vi "AlliGator Save Phasor Plot Additional Data.vi"(4 "Save only if selected":bool, 5 "Intensity Weighted ? (F)":bool, 6 "Save as...":bool, 7 "Phasor Plot Folder Path (empty)":path, 8 "error in (no error)":errorcluster, 9 "Raw Phasor Plot":T1={"Phasor Plot Name"="", "Raw Phasor Plot"=[], "Phasor Frequency"=160000000.0, "[Decay Metadata]"=[], "Raw Phasor Plot SDV"=[], "Phasor SDV Options"={"Compute Estimated SDV"=FALSE, "# Replicas"=100, "Use Estimated Average Phasor"=FALSE}, "[Calibration Phasor]"=[], "Intensity Array"=[]} {"[Decay Metadata]"."# Folds" min=1; "[Decay Metadata]"."ROI Descriptor"."Contours"."Type" items=["No Selection", "Point", "Line", "Rectangle", "Oval", "Polygon", "Freehand Region", "Annulus", "Unused2", "Unused3", "Broken Line", "Freehand Line", "Rotated Rectangle"]}, 10 "Selected Plot":i32, 11 "Phasor Graph":refnum<vi>) -> (0 "Error Out":errorcluster, 1 "Message":string)   [LabVIEW 2021, in "AlliGator Phasor Graph.lvlib"]
doc: "Save the user-selected Phasor Plot additional data."
uses:
  AlliGator Phasor Graph.lvlib
  AlliGator Raw Phasor Plot Data v5.ctl
  Phasor/Phasor (g, s).ctl
  AlliGator Decay Metadata v3.ctl
  Decay Analysis/Decay Preprocessing/AlliGator Decay Background Subtraction Info.ctl
  Decay Analysis/Decay Preprocessing/AlliGator Baseline Subtraction Method.ctl
  Graphs/XY Graph/XY Graph Plot Shift Parameters.ctl
  Graphs/XY Graph/XY Graph Plot Shift Method.ctl
  Decay Analysis/Decay Preprocessing/AlliGator Decay Extrapolation Parameters.ctl
  Phasor/Phasor Standard Deviation Options.ctl
  Phasor/Calibration Phasor (m, phi).ctl
  Phasor/Phasor.lvlib
  Decay Analysis/Decay Preprocessing/AlliGator Decay Preprocessing.lvlib
  Graphs/XY Graph/XY Graph Add-Ons.lvlib
panel:
  # "see the AlliGator License on the block diagram (Ctrl+E or Window:Show Block Diagram)"
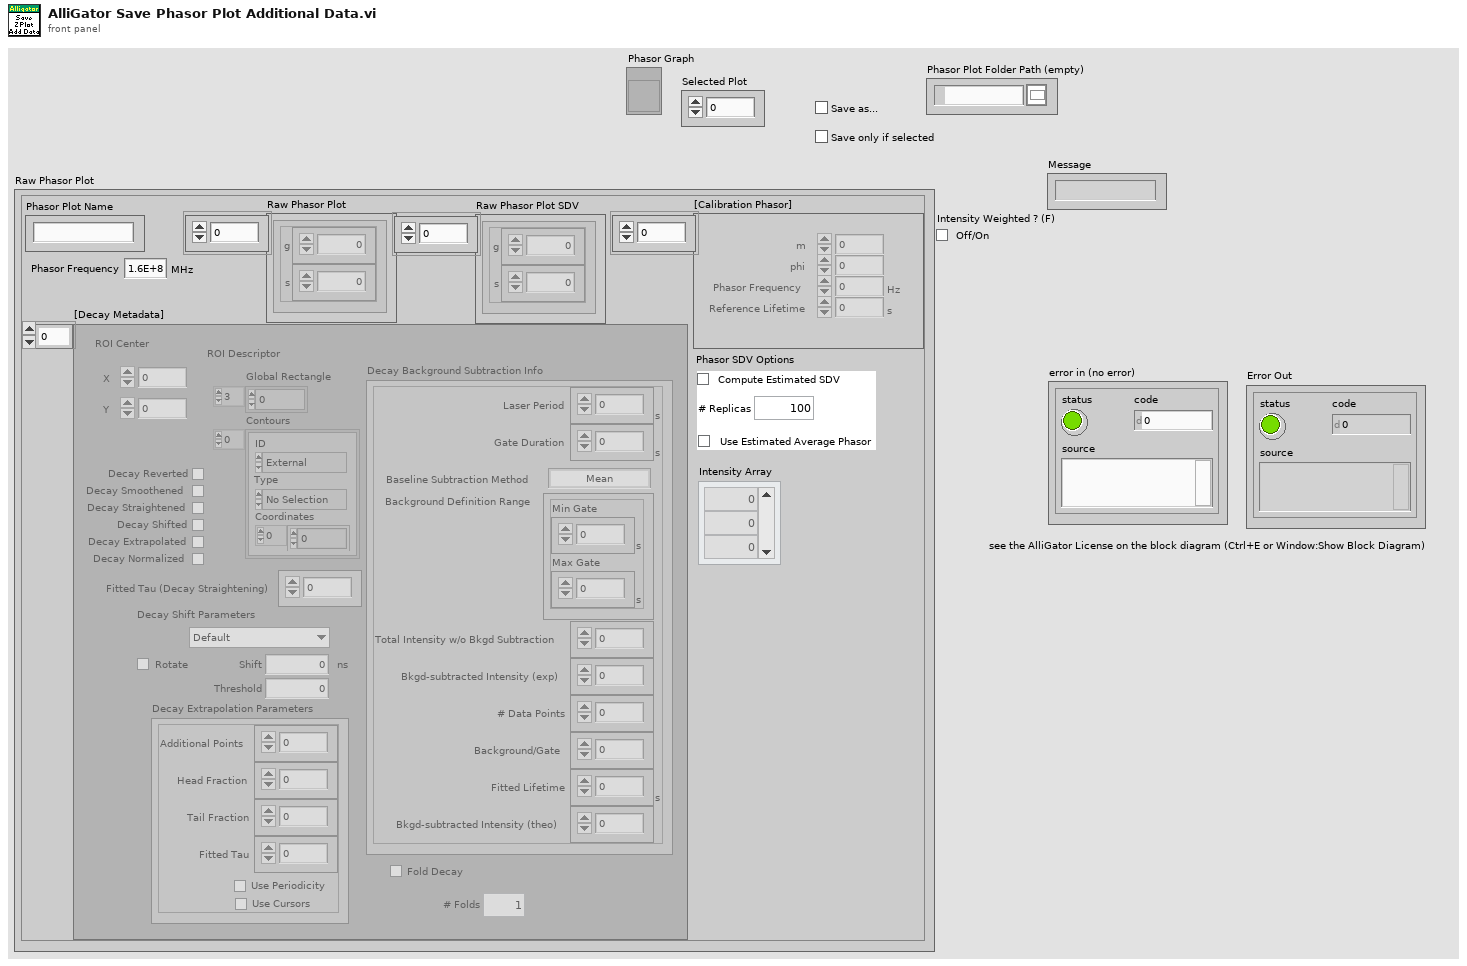
[diagram p1: front panel]
types:
  T1 = typedef "AlliGator Phasor Graph.lvlib/AlliGator Raw Phasor Plot Data v5.ctl" = cluster{"Phasor Plot Name":string, "Raw Phasor Plot":T2[], "Phasor Frequency":dbl[unit], "[Decay Metadata]":T3[], "Raw Phasor Plot SDV":T2[], "Phasor SDV Options":T10, "[Calibration Phasor]":T11[], "Intensity Array":dbl[]}
  T2 = typedef "Phasor.lvlib/Phasor (g, s).ctl" = cluster{"g":dbl, "s":dbl}
  T3 = typedef "AlliGator Phasor Graph.lvlib/AlliGator Decay Metadata v3.ctl" = cluster{"ROI Descriptor":T4, "ROI Center":cluster{"X":i32, "Y":i32}, "Decay Background Subtraction Info":T5, "Decay Reverted":bool, "Decay Smoothened":bool, "Decay Straightened":bool, "Fitted Tau (Decay Straightening)":dbl, "Decay Shift Parameters":T7, "Decay Shifted":bool, "Decay Extrapolated":bool, "Decay Extrapolation Parameters":T9, "Decay Normalized":bool, "Fold Decay":bool, "# Folds":u32}
  T4 = typedef "ROI Descriptor" = cluster{"Global Rectangle":i32[], "Contours":cluster{"ID":enum32{"External", "Internal"}, "Type":u32, "Coordinates":i32[]}[]}
  T5 = typedef "AlliGator Decay Preprocessing.lvlib/AlliGator Decay Background Subtraction Info.ctl" = cluster{"Laser Period":dbl[unit], "Gate Duration":dbl[unit], "Baseline Subtraction Method":T6, "Background Definition Range":cluster{"Min Gate":dbl[unit], "Max Gate":dbl[unit]}, "Total Intensity w/o Bkgd Subtraction":dbl, "Bkgd-subtracted Intensity (exp)":dbl, "# Data Points":i32, "Background/Gate":dbl, "Fitted Lifetime":dbl[unit], "Bkgd-subtracted Intensity (theo)":dbl}
  T6 = typedef "AlliGator Decay Preprocessing.lvlib/AlliGator Baseline Subtraction Method.ctl" = enum16{"Mean", "Min", "Square Gated Single-Exponential", "File", "Constant"}
  T7 = typedef "XY Graph Add-Ons.lvlib/XY Graph Plot Shift Parameters.ctl" = cluster{"Type":T8, "Shift":dbl[unit], "Threshold":dbl, "Rotate":bool}
  T8 = typedef "XY Graph Add-Ons.lvlib/XY Graph Plot Shift Method.ctl" = enum16{"Default", "CFD", "Threshold", "Cross-Correlation"}
  T9 = typedef "AlliGator Decay Preprocessing.lvlib/AlliGator Decay Extrapolation Parameters.ctl" = cluster{"Additional Points":u32, "Head Fraction":dbl, "Fitted Tau":dbl, "Use Periodicity":bool, "Use Cursors":bool, "Tail Fraction":dbl}
  T10 = typedef "Phasor.lvlib/Phasor Standard Deviation Options.ctl" = cluster{"Compute Estimated SDV":bool, "# Replicas":u32, "Use Estimated Average Phasor":bool}
  T11 = typedef "Phasor.lvlib/Calibration Phasor (m, phi).ctl" = cluster{"m":dbl, "phi":dbl, "Phasor Frequency":dbl[unit], "Reference Lifetime":dbl[unit]}
  T12 = typedef "AlliGator Phasor Graph.lvlib/AlliGator Phasor Plot Exported Data Selection.ctl" = cluster{"x":bool, "y":bool, "g":bool, "s":bool, "phi":bool, "m":bool, "tau phi":bool, "tau m":bool, "phasor ratio (intensity-weighted)":bool, "<tau> (intensity-weighted)":bool, "phasor ratio (amplitude-weighted)":bool, "<tau> (amplitude-weighted)":bool, "g SDV":bool, "s SDV":bool, "phi SDV":bool, "m SDV":bool, "tau phi SDV":bool, "tau m SDV":bool, "phasor ratio (intensity-weighted) SDV":bool, "<tau> (intensity-weighted) SDV":bool, "phasor ratio (amplitude-weighted) SDV":bool, "<tau> (amplitude-weighted) SDV":bool, "Intensity":bool}
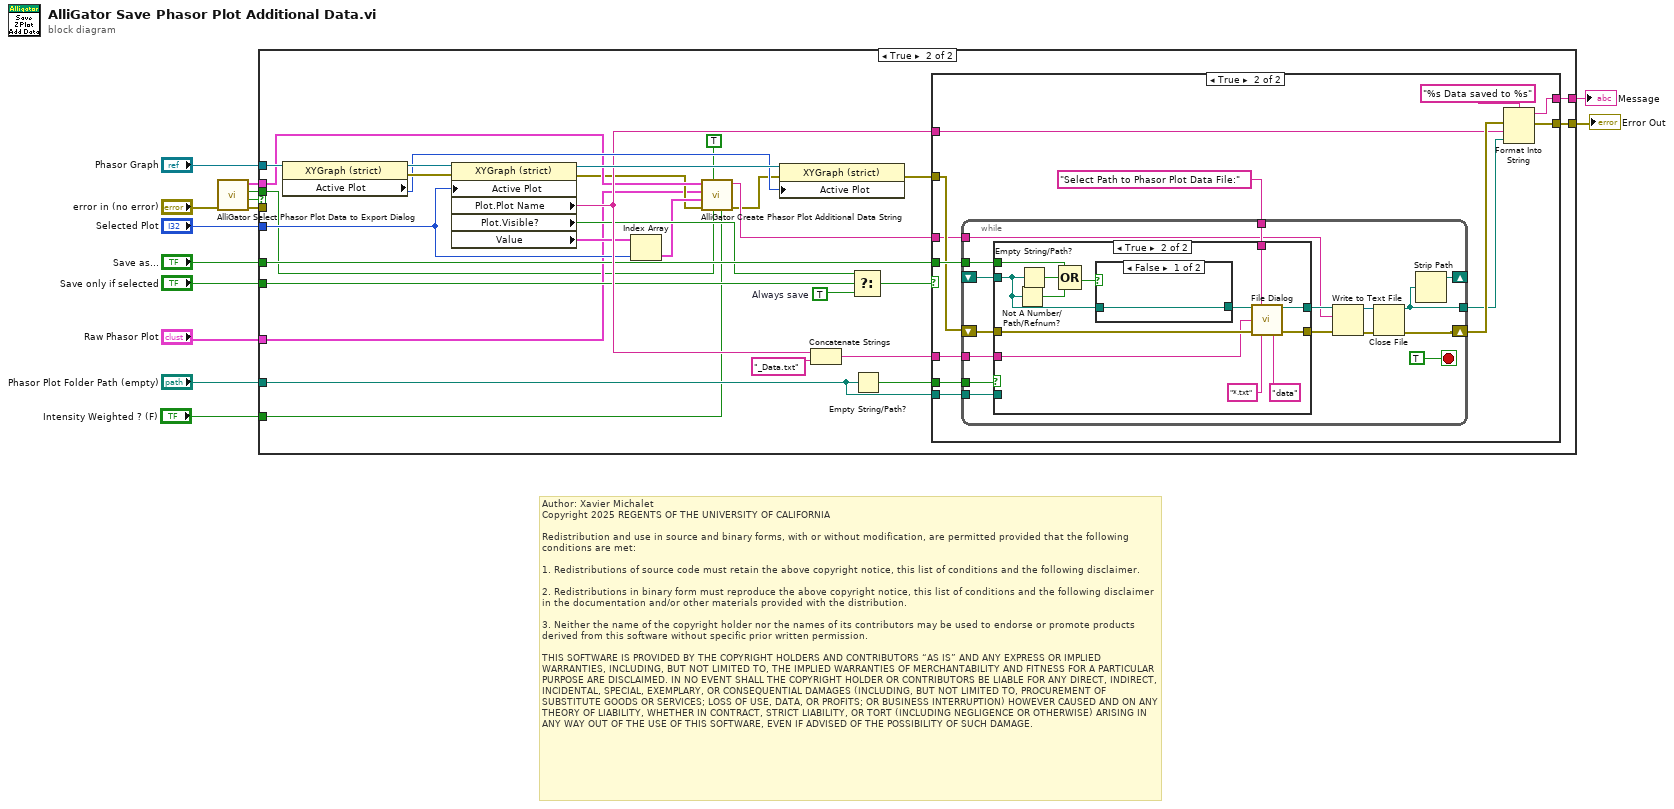
[diagram p0: block diagram]
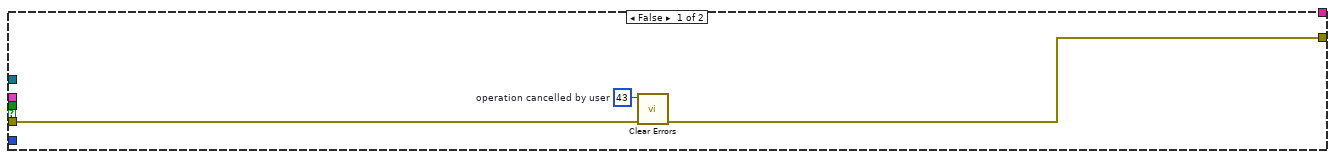
[diagram p2: hidden frame]
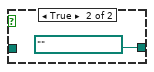
[diagram p5: hidden frame]
diagram:
  # "Author: Xavier Michalet\nCopyright 2025 REGENTS OF THE UNIVERSITY OF CALIFORNIA\n\nRedistribution and use in source and binary forms, with or without modification, are permitted provided that the following conditions are met:\n\n1. Redistributions of source code must retain the above copyright notice, this list of conditions and the following disclaimer.\n\n2. Redistributions in binary form must reproduce the above copyright notice, this list of conditions and the following disclaimer in the documentation and/or other materials provided with the distribution.\n\n3. Neither the name of the copyright holder nor the names of its contributors may be used to endorse or promote products derived from this software without specific prior written permission.\n\nTHIS SOFTWARE IS PROVIDED BY THE COPYRIGHT HOLDERS AND CONTRIBUTORS “AS IS” AND ANY EXPRESS OR IMPLIED WARRANTIES, INCLUDING, BUT NOT LIMITED TO, THE IMPLIED WARRANTIES OF MERCHANTABILITY AND FITNESS FOR A PARTICULAR PURPOSE ARE DISCLAIMED. IN NO EVENT SHALL THE COPYRIGHT HOLDER OR CONTRIBUTORS BE LIABLE FOR ANY DIRECT, INDIRECT, INCIDENTAL, SPECIAL, EXEMPLARY, OR CONSEQUENTIAL DAMAGES (INCLUDING, BUT NOT LIMITED TO, PROCUREMENT OF SUBSTITUTE GOODS OR SERVICES; LOSS OF USE, DATA, OR PROFITS; OR BUSINESS INTERRUPTION) HOWEVER CAUSED AND ON ANY THEORY OF LIABILITY, WHETHER IN CONTRACT, STRICT LIABILITY, OR TORT (INCLUDING NEGLIGENCE OR OTHERWISE) ARISING IN ANY WAY OUT OF THE USE OF THIS SOFTWARE, EVEN IF ADVISED OF THE POSSIBILITY OF SUCH DAMAGE."
  n1 = call "AlliGator Select Phasor Plot Data to Export Dialog.vi"("error in (no error)"="error in (no error)") -> ("error out"=w6:errorcluster, "OK?"=w5:bool, "Average Plot Data"=w3:bool, "Phasor Plot Exported Data"=w4:T12)  [unwired: 7 in]
  n2 = case shown="True" w5 {
    tunnel: "Phasor Graph" -> [_ w46]
    tunnel: "Selected Plot" -> [_ w26]
    tunnel: [w16 w41] -> w12
    tunnel: "Raw Phasor Plot" -> [_ w22]
    tunnel: "Save as..." -> [_ w36]
    tunnel: "Phasor Plot Folder Path (empty)" -> [_ w34]
    tunnel: "Save only if selected" -> [_ w33]
    tunnel: w6 -> [w17 _]
    tunnel: w4 -> [_ w28]
    tunnel: w3 -> [_ w21]
    tunnel: [_ w19] -> w2
    tunnel: "Intensity Weighted ? (F)" -> [_ w18]
    frame False {
      w15 = 43  # operation cancelled by user
      n3 = call <vilib>:"Clear Errors.vi"("error in (no error)"=w17, "specific error code to clear (0: all)"=w15) -> ("error out"=w16:errorcluster)  [unwired: 4 in, 1 out]
    }
    frame True {
      w32 = TRUE  # Always save
      n4 = property class="XYGraph (strict)"(reference=w46) -> (reference out=w45:refnum<vi>, error out=w44:errorcluster, "Active Plot"=w42:u32)  [unwired: 1 in]
      n5 = property class="XYGraph (strict)"(reference=w45, error in=w44, "Active Plot"=w26) -> (reference out=w43:refnum<vi>, error out=w24:errorcluster, "Plot.Plot Name"=w40:string, "Plot.Visible?"=w31:bool, "Value"=w27:cluster{dbl[], dbl[]}[])
      n6 = Index Array(array=w27, index=w26) -> (element=w25:cluster{dbl[], dbl[]})
      n7 = call "AlliGator Create Phasor Plot Additional Data String.vi"("Intensity Weighted ? (F)"=w18, "Average Plot Data (F)"=w21, "Include Header String (F)"=TRUE ("Include Headre  String"), "error in (no error)"=w24, "Calibrated Phasor Plot"=w25, "Raw Phasor Plot"=w22, "Phasor Plot Exported Data"=w28) -> ("error out"=w23:errorcluster, "Phasor Plot Additional Data String"=w29:string)  [unwired: 3 in]
      n8 = property class="XYGraph (strict)"(reference=w43, error in=w23, "Active Plot"=w42) -> (error out=w37:errorcluster)  [unwired: 1 out]
      n9 = Concatenate Strings(w40, "_Data.txt" ("string")) -> (w38:string)
      n10 = Select(t=w31, s=w33, f=w32) -> (s? t:f=w30:bool)
      n11 = Empty String/Path?(string/path=w34) -> (empty?=w35:bool)
      n12 = case shown="True" w30 {
        tunnel: [w47 w48] -> w41
        tunnel: w40 -> [_ w57]
        tunnel: w38 -> [_ w55]
        tunnel: w37 -> [w47 w51]
        tunnel: w36 -> [_ w54]
        tunnel: w35 -> [_ w53]
        tunnel: w34 -> [_ w52]
        tunnel: w29 -> [_ w50]
        tunnel: [_ w49] -> w19
        frame False {
        }
        frame True {
          n13 = while {
            tunnel: w50 -> [w67]
            tunnel: [w63] -> w58
            shift-right: [w64] -> w59
            shift-left: w51 -> [w71]
            shift-right: [w76] -> _
            shift-left: _ -> [w73]
            tunnel: w54 -> [w74]
            tunnel: "Select Path to Phasor Plot Data File:" ("Prompt") -> [w72]
            tunnel: w55 -> [w70]
            tunnel: w53 -> [w62]
            tunnel: w52 -> [w61]
            stop <- TRUE stop-if-true
            n14 = case shown="True" w62 {
              tunnel: w74 -> [_ w89]
              tunnel: w73 -> [_ w87]
              tunnel: w72 -> [_ w85]
              tunnel: w71 -> [w77 w84]
              tunnel: w70 -> [_ w81]
              tunnel: [w78 w80] -> w69
              tunnel: [w77 w79] -> w68
              tunnel: w61 -> [w78 _]
              frame False {
              }
              frame True {
                n15 = Not A Number/Path/Refnum?(number/path/refnum=w87) -> (NaN/Path/Refnum?=w90:bool)
                n16 = Empty String/Path?(string/path=w87) -> (empty?=w91:bool)
                n17 = Compound Arithmetic op=OR(w89, w91, w90) -> (w88:bool)
                n18 = case shown="False" w88 {
                  tunnel: [w92 path "" ("start path  (Not A Path)")] -> w86
                  tunnel: w87 -> [w92 _]
                  frame False {
                  }
                  frame True {
                  }
                }
                n19 = call "File Dialog"("start path"=w86, "prompt"=w85, "default name"=w81, "error in"=w84, "pattern (all files)"="*.txt" ("Pattern (*.xml;*.XML)"), "pattern label"="data" ("File Extension (xml)")) -> ("selected path"=w80:path, "error out"=w79:errorcluster)  [unwired: 6 in, 2 out]
              }
            }
            n20 = Write to Text File(file (use dialog)=w69, text=w67, error in=w68) -> (refnum out=w66:refnum<file>, error out=w65:errorcluster)  [unwired: 1 in, 1 out]
            n21 = Close File(refnum=w66, error in=w65) -> (path=w63:path, error out=w64:errorcluster)
            n22 = Strip Path(path=w63) -> (stripped path=w76:path)  [unwired: 1 out]
          }
          n23 = Format Into String(format string="%s Data saved to %s", error in=w59, w57, w58) -> (resulting string=w49:string, error out=w48:errorcluster)  [unwired: 1 in]
        }
      }
    }
  }
  "Error Out" <- w12
  "Message" <- w2
